vi "Read Data.vi"(8 "error in (no error)":errorcluster, 11 "FlipMir in":refnum<class "FlipMir.lvclass">) -> (0 "error out":errorcluster, 1 "Time Stamp":timestamp, 2 "Status":bool, 3 "FlipMir out":refnum<class "FlipMir.lvclass">)   [LabVIEW 2016, in "FlipMir.lvclass"]
uses:
  FlipMir.lvclass
  FlipMir.lvclass/FlipMir.ctl
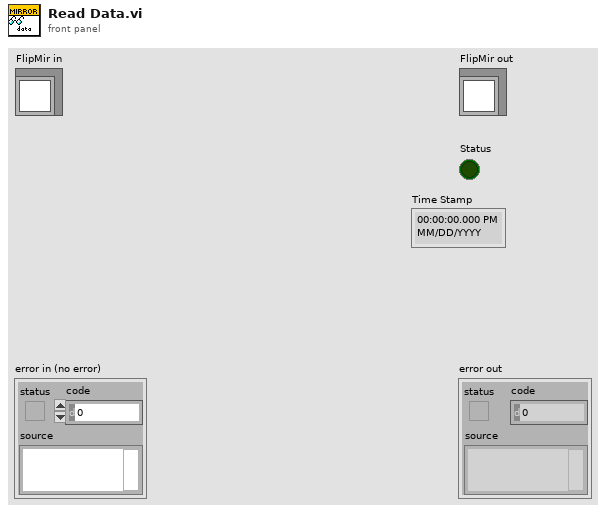
[diagram p1: front panel]
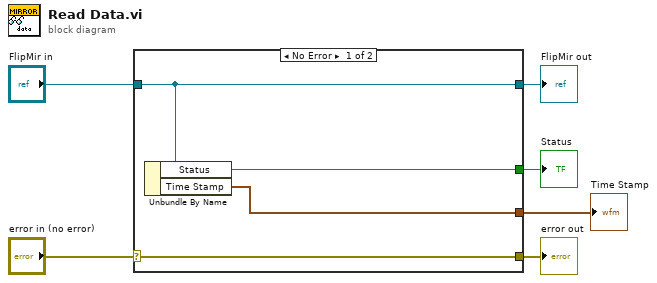
[diagram p0: block diagram]
diagram:
  n1 = case shown="No Error" "error in (no error)" {
    selector: "error in (no error)" -> [w10 w11]
    tunnel: [w10 w11] -> w5
    tunnel: [w9 w12] -> w3
    tunnel: "FlipMir in" -> [w9 w12]
    tunnel: [w8 _] -> w2
    tunnel: [w7 _] -> w1
    frame No Error {
      n2 = Unbundle By Name(w9) -> ("Status"=w8:bool, "Time Stamp"=w7:timestamp)
    }
    frame Error {
    }
  }
  "error out" <- w5
  "FlipMir out" <- w3
  "Status" <- w2
  "Time Stamp" <- w1
